vi "ЛР2 защита Грамотин.vi"() -> ()   [LabVIEW 2012]
uses:
  <vilib>/Analysis/NI_AALPro.lvlib
  <vilib>/Analysis/2dsp.llb/Real FFT.vi
panel:
  out "Phase":cluster{"y":dbl, dbl, dbl[]}(graph)
  out "Amplitude":cluster{"y":dbl, dbl, dbl[]}(graph)
  out "DC":dbl
  out "RMS 2":dbl
  out "Minimum":dbl
  out "Maximum":dbl
  in  "Cluster":cluster{" n":dbl, "k":dbl, "m":dbl, "N":i32} {"m" scale=0.0..10.0; "k" scale=-10.0..10.0; "n" scale=0.0..100.0}
  out "Waveform Graph":dbl[](graph)
  out "Waveform Chart 2":dbl[](graph)
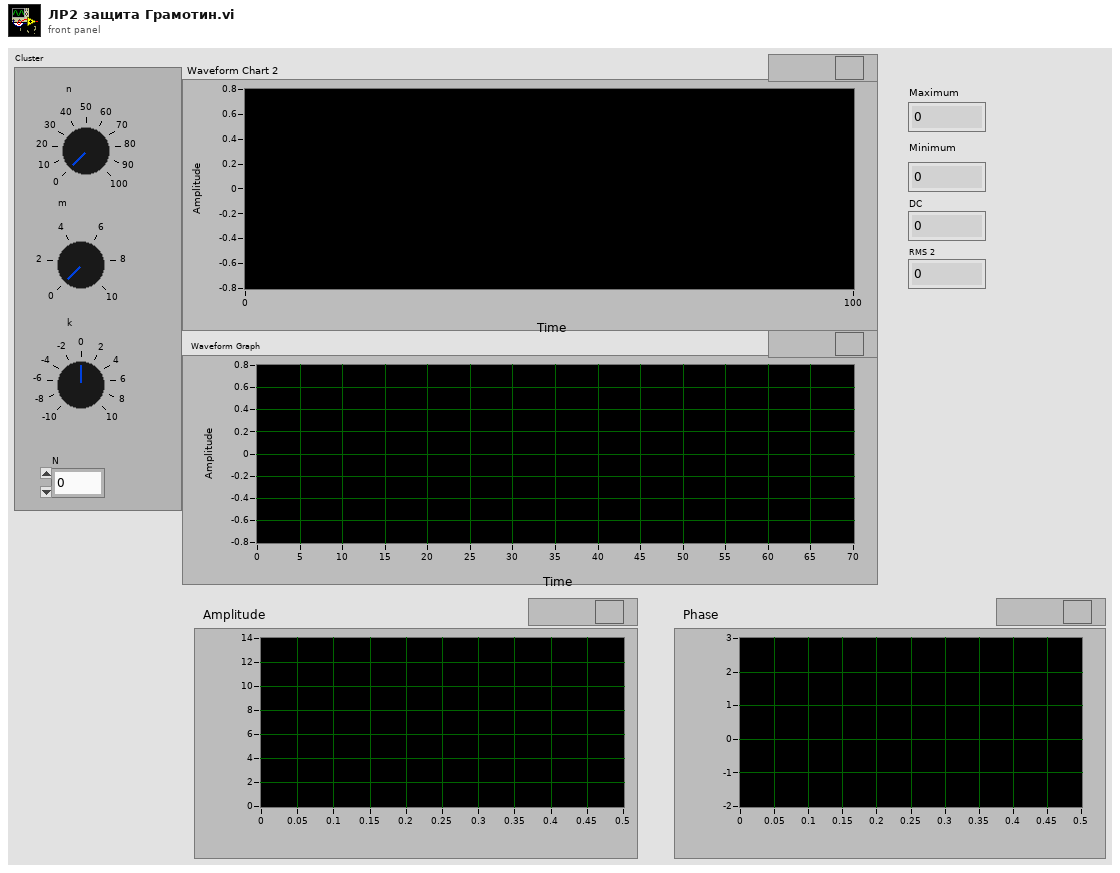
[diagram p1: front panel]
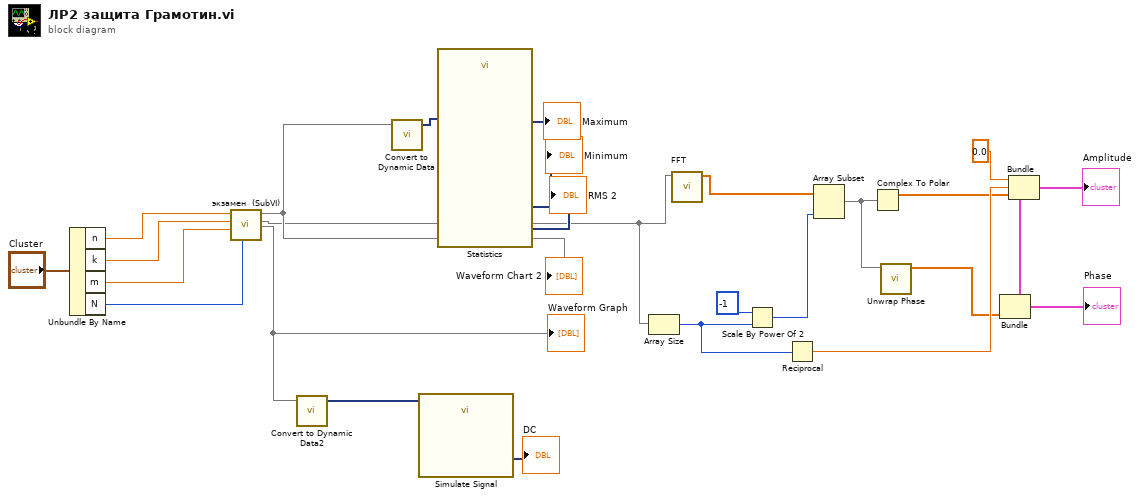
[diagram p0: block diagram]
diagram:
  n1 = Unbundle By Name "Unbundle By Name"("Cluster") -> ("n"=w24:dbl, "k"=w23:dbl, "m"=w22:dbl, "N"=w21:i32)
  n2 = call "экзамен  (SubVI).vi"("N"=w21, "C"=w22, "B"=w23, "A"=w24) -> (2:w6, 3:w17)  [unwired: 6 in]
  "Waveform Chart 2" <- w17
  "Waveform Graph" <- w6
  n3 = call "Convert to Dynamic Data2"("Array"=w6) -> ("Dynamic Data Type"=w14:dynamicdata)  [unwired: 3 in]
  n4 = call "Convert to Dynamic Data"("Array"=w17) -> ("Dynamic Data Type"=w20:dynamicdata)  [unwired: 3 in]
  n5 = call "Simulate Signal"("Offset"=w14) -> ("DC"=→"DC":dynamicdata)  [unwired: 13 in, 1 out]
  n6 = call "Statistics"("Signals"=w20) -> ("RMS"=→"RMS 2":dynamicdata, "Minimum"=→"Minimum":dynamicdata, "Maximum"=→"Maximum":dynamicdata)  [unwired: 23 in, 1 out]
  n7 = Array Size(array=w6) -> (size(s)=w13:i32)
  n8 = call-poly <vilib>:"FFT.vi"("X"=w6) -> ("FFT {X}"=w11:cdb[])  [unwired: 9 in, 1 out]
  n9 = Scale By Power Of 2(n=i16 -1, x=w13) -> (x*2^n=w10:i32)
  n10 = Reciprocal(x=w13) -> (1/x=w8:dbl)
  n11 = Array Subset "Array Subset"(array=w11, length=w10) -> (w9:cdb[])  [unwired: 1 in]
  n12 = Complex To Polar(r * e^(i*theta)=w9) -> (r=w4:dbl[])  [unwired: 1 out]
  n13 = call <vilib>:"Unwrap Phase.vi"("Phase"=w9) -> ("Unwrapped Phase"=w5:dbl[])  [unwired: 9 in, 1 out]
  n14 = Bundle "Bundle"("y"=0.0, w8, w4) -> (w1:cluster{"y":dbl, dbl, dbl[]})  [unwired: 1 in]
  "Amplitude" <- w1
  n15 = Bundle "Bundle"(cluster=w1, w5) -> (→"Phase":cluster{"y":dbl, dbl, dbl[]})  [unwired: 2 in]
